vi "Filter.vi"(8 "error in (no error)":errorcluster, 10 "Selected Runnables":string[](array[string]), 11 "LUnit Test Suite In":refnum<class "LUnit Test Suite.lvclass">) -> (0 "error out":errorcluster, 3 "LUnit Test Suite Out":refnum<class "LUnit Test Suite.lvclass">)   [LabVIEW 2020, in "LUnit Test Suite.lvclass"]
doc: "Select which tests are active. This applies recursively to nested suites."
uses:
  LUnit Test Suite.lvclass
  C:/git/astemes-lunit/source/Runnable.lvclass
  LUnit Test Suite.lvclass/LUnit Test Suite.ctl
  <vilib>/Utility/miscctls.llb/LVMapReplaceAction.ctl
  Runnable.lvclass
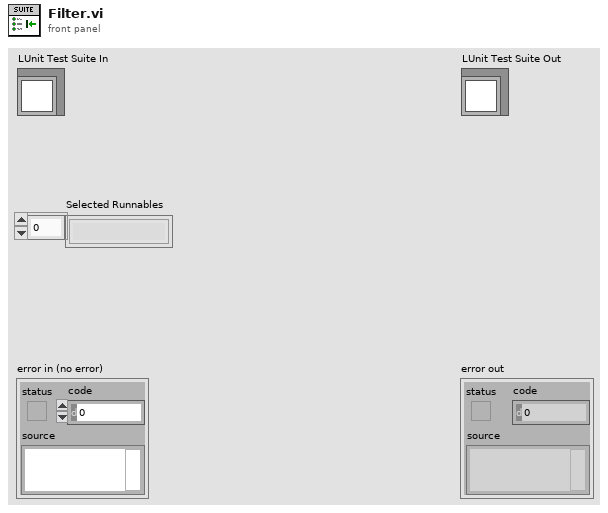
[diagram p1: front panel]
types:
  T1 = typedef "LVMapReplaceAction.ctl" = enum32{"Modify Entry only if found", "Add or Modify Entry", "Delete Entry"}
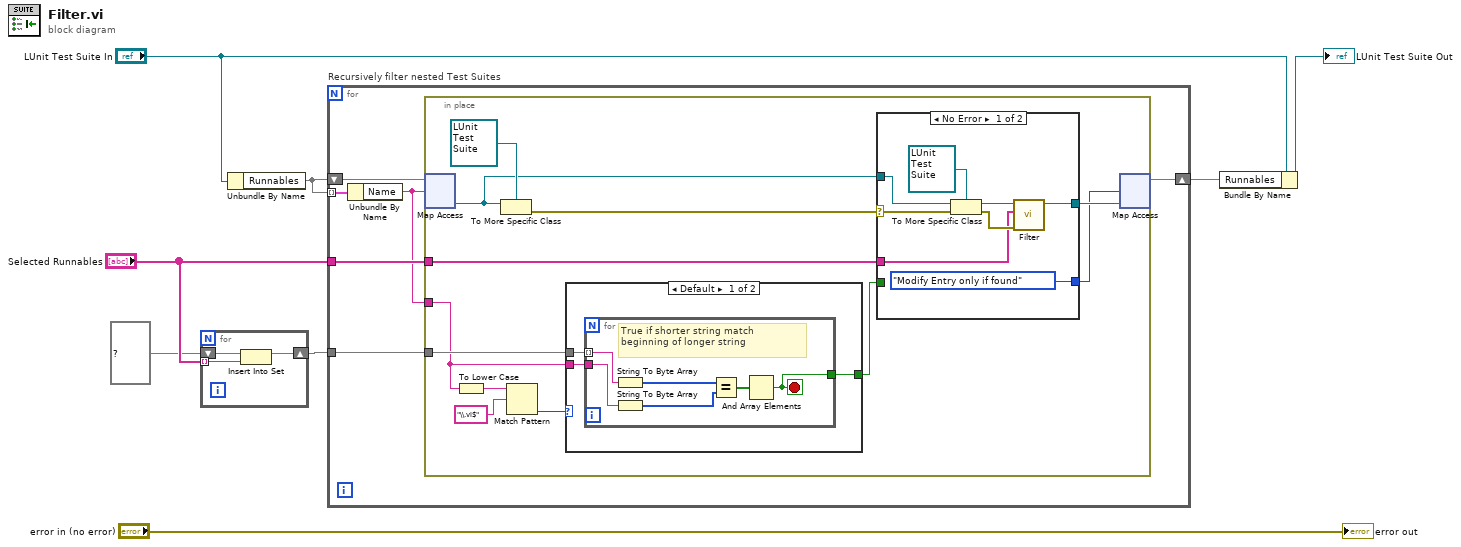
[diagram p0: block diagram]
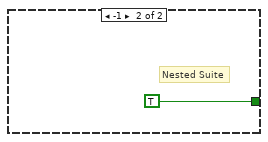
[diagram p2: hidden frame]
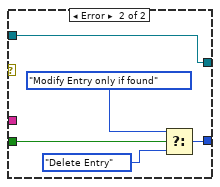
[diagram p3: hidden frame]
diagram:
  n1 = for {
    shift-right: [w10] -> w1
    shift-left: set{string} {} ("set") -> [w11]
    tunnel: "Selected Runnables" -> [w9] mode=indexing
    n2 = Insert Into Set(10:w9, 11:w11) -> (3:w10:set{string})  [unwired: 1 out]
  }
  n3 = Unbundle By Name("LUnit Test Suite In") -> ("Runnables"=w3:map{string, refnum<class "Runnable.lvclass">})
  n4 = for "Recursively filter nested Test Suites" {
    shift-right: [w16] -> w2
    shift-left: w3 -> [w17]
    tunnel: w3 -> [w14] mode=indexing
    tunnel: "Selected Runnables" -> [w15]
    tunnel: w1 -> [w13]
    n5 = Unbundle By Name(w14) -> ("Name"=w12:string)
    n6 = in-place {
      in-place-border: w15 -> [w25]
      in-place-border: w13 -> [w24]
      in-place-border: w12 -> [w23]
      n7 = in-place-map #1(w17, w12) -> (w27:refnum<class "Runnable.lvclass">)  [unwired: 1 in, 1 out]
      n8 = To Lower Case(string=w23) -> (all lower case string=w20:string)
      n9 = To More Specific Class(target class=refnum<class "LUnit Test Suite.lvclass"> refnum ("LUnit Test Suite V2.lvclass"), reference=w27) -> (error out=w28:errorcluster)  [unwired: 1 in, 1 out]
      n10 = Match Pattern(string=w20, regular expression="\\.vi$") -> (offset past match=w19:i32)  [unwired: 1 in, 3 out]
      n11 = case shown="Default" w19 {
        tunnel: w24 -> [w32 _]
        tunnel: [w31 TRUE] -> w22
        tunnel: w23 -> [w30 _]
        frame Default {
          n12 = for {
            tunnel: w32 -> [w38] mode=indexing
            tunnel: w30 -> [w37]
            tunnel: [w33] -> w31
            stop <- w33 stop-if-true
            # "True if shorter string match beginning of longer string"
            n13 = String To Byte Array(string=w38) -> (unsigned byte array=w36:u8[])
            n14 = String To Byte Array(string=w37) -> (unsigned byte array=w35:u8[])
            n15 = Equal?(x=w36, y=w35) -> (x = y?=w34:bool[])
            n16 = And Array Elements(Boolean array=w34) -> (logical AND=w33:bool)
          }
        }
        frame -1 {
          # "Nested Suite"
        }
      }
      n17 = case shown="No Error" w28 {
        selector: w28 -> [w45 _]
        tunnel: w27 -> [w46 w52]
        tunnel: [w42 w52] -> w26
        tunnel: w25 -> [w41 _]
        tunnel: w22 -> [_ w51]
        tunnel: [LVMapReplaceAction."Modify Entry only if found" ("action") w50] -> w21
        frame No Error {
          n18 = To More Specific Class(target class=refnum<class "LUnit Test Suite.lvclass"> refnum ("LUnit Test Suite V2.lvclass"), reference=w46, error in=w45) -> (specific class reference=w44:refnum<class "LUnit Test Suite.lvclass">, error out=w43:errorcluster)
          n19 = call "Filter.vi"("error in (no error)"=w43, "Selected Runnables"=w41, "LUnit Test Suite In"=w44) -> ("LUnit Test Suite Out"=w42:refnum<class "LUnit Test Suite.lvclass">)  [unwired: 7 in, 1 out]
        }
        frame Error {
          n20 = Select(t=LVMapReplaceAction."Modify Entry only if found" ("action"), s=w51, f=LVMapReplaceAction."Delete Entry" ("action")) -> (s? t:f=w50:T1)
        }
      }
      n21 = in-place-map #1(w26, w21) -> (w16:map{string, refnum<class "Runnable.lvclass">})  [unwired: 2 out]
    }
  }
  n22 = Bundle By Name(cluster="LUnit Test Suite In", "Runnables"=w2) -> (→"LUnit Test Suite Out":refnum<class "LUnit Test Suite.lvclass">)
  "error out" <- "error in (no error)"
